vi "RemoveSelfFromNameList.vi"(9 "self Name":string, 10 "Names in use":string[](array[string])) -> (2 "Reserved Names":string[](array[string]))   [LabVIEW 2013]
doc: "Remove \"self Name\" from \"Names in Use\" returning the reserved names which \"self\" cannot use."
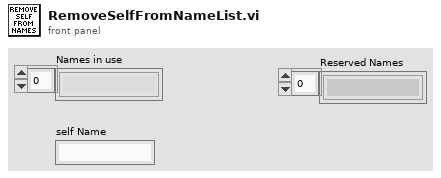
[diagram p1: front panel]
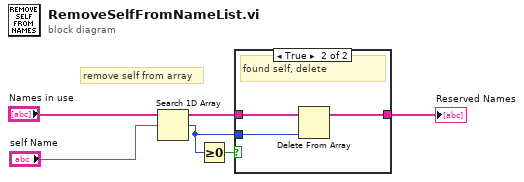
[diagram p0: block diagram]
diagram:
  # "remove self from array"
  n1 = Search 1D Array(1D array="Names in use", element="self Name") -> (index of element=w5:i32)  [unwired: 1 in]
  n2 = Greater Or Equal To 0?(x=w5) -> (x >= 0?=w4:bool)
  n3 = case shown="True" w4 {
    tunnel: "Names in use" -> [w6 w9]
    tunnel: w5 -> [_ w8]
    tunnel: [w6 w7] -> w2
    frame False {
      # "did not find self"
    }
    frame True {
      # "found self, delete"
      n4 = Delete From Array(array=w9, index=w8) -> (array with subset deleted=w7:string[])  [unwired: 1 in, 1 out]
    }
  }
  "Reserved Names" <- w2
